vi "Drive Teleop.vi"(8 "CargoAlign?":bool, 9 "SlowMode?":bool, 10 "Wheel":dbl, 11 "Throttle":dbl) -> ()   [LabVIEW 2020]
uses:
  <vilib>/Rock Robotics/Network Tables/NT Read Number.vi
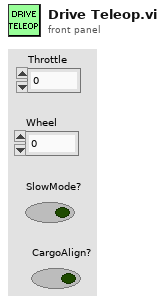
[diagram p1: front panel]
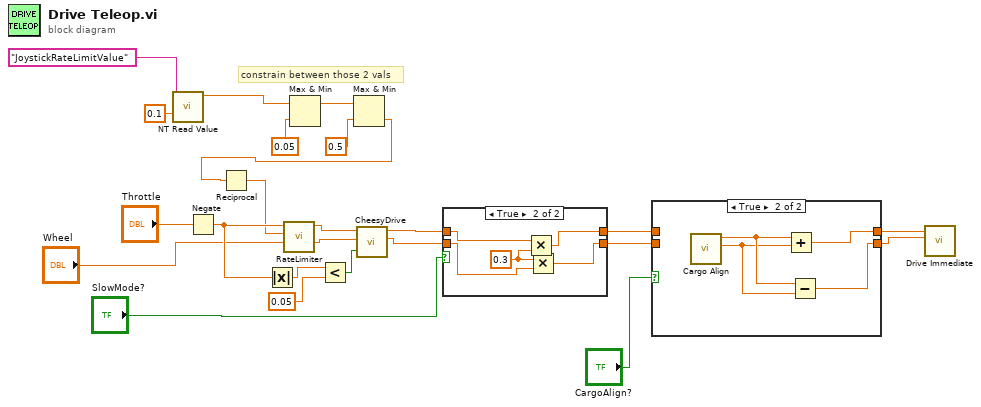
[diagram p0: block diagram]
diagram:
  # "constrain between those 2 vals"
  n1 = call-poly <vilib>:"NT Read Value.vi"("Default Value"=0.1, "Name"="JoystickRateLimitValue") -> ("Numeric"=w11:dbl)  [unwired: 8 in, 1 out]
  n2 = Negate(x="Throttle") -> (-x=w20:dbl)
  n3 = Absolute Value(x=w20) -> (abs(x)=w23:dbl)
  n4 = Max & Min(x=w11, y=0.05) -> (max(x,y)=w10:dbl)  [unwired: 1 out]
  n5 = Less?(x=w23, y=0.05) -> (x < y?=w21:bool)
  n6 = Max & Min(x=w10, y=0.5) -> (min(x,y)=w9:dbl)  [unwired: 1 out]
  n7 = Reciprocal(x=w9) -> (1/x=w18:dbl)
  n8 = call "RateLimiter.vi"("Max dx/dt"=w18, "Input"=w20) -> ("Output"=w19:dbl)  [unwired: 9 in]
  n9 = call "CheesyDrive.vi"("Quickturn"=w21, "Wheel"="Wheel", "Throttle"=w19) -> ("Right PWM"=w16:dbl, "Left PWM"=w17:dbl)  [unwired: 7 in]
  n10 = case shown="True" "SlowMode?" {
    tunnel: [w25 w27] -> w5
    tunnel: w17 -> [w25 w29]
    tunnel: w16 -> [w24 w28]
    tunnel: [w24 w26] -> w4
    frame False {
    }
    frame True {
      w30 = 0.3
      n11 = Multiply(x=w29, y=w30) -> (x*y=w27:dbl)
      n12 = Multiply(x=w30, y=w28) -> (x*y=w26:dbl)
    }
  }
  n13 = case shown="True" "CargoAlign?" {
    tunnel: w5 -> [w32 _]
    tunnel: w4 -> [w31 _]
    tunnel: [w32 w36] -> w3
    tunnel: [w31 w33] -> w2
    frame False {
    }
    frame True {
      n14 = call "Cargo Align.vi"() -> ("Wheel"=w34:dbl, "Throttle"=w35:dbl)  [unwired: 10 in]
      n15 = Add(x=w35, y=w34) -> (x+y=w36:dbl)
      n16 = Subtract(x=w35, y=w34) -> (x-y=w33:dbl)
    }
  }
  n17 = call "Drive Immediate.vi"("Right Setpoint"=w2, "Left Setpoint"=w3) -> ()  [unwired: 9 in, 1 out]
